vi "LabJSONExample.vi"(8 "Error In":errorcluster, 9 "Settings":T1, 10 "JSON Input":string="{\n  \"Cluster\":{\n    \"Numeric\":1,\n    \"String\":\"One\",\n    \"Checkbox\":false\n  },\n  \"Array - String\":[[]],\n  \"Numeric\":0,\n  \"File Path Control\":\"\",\n  \"Checkbox\":false\n}", 11 "VI Path":path=path "Sample/SampleVI.vi") -> (0 "Error Out":errorcluster, 3 "JSON Output":string)   [LabVIEW 2019, in "LabJSON.lvlib"]
doc: "Take JSON as input, run the VI, and return the output as JSON"
uses:
  LabJSON.lvlib
  Typedefs/Settings.ctl
  <vilib>/SLL Toolkit/SLL File IO/SLL File IO.lvlib
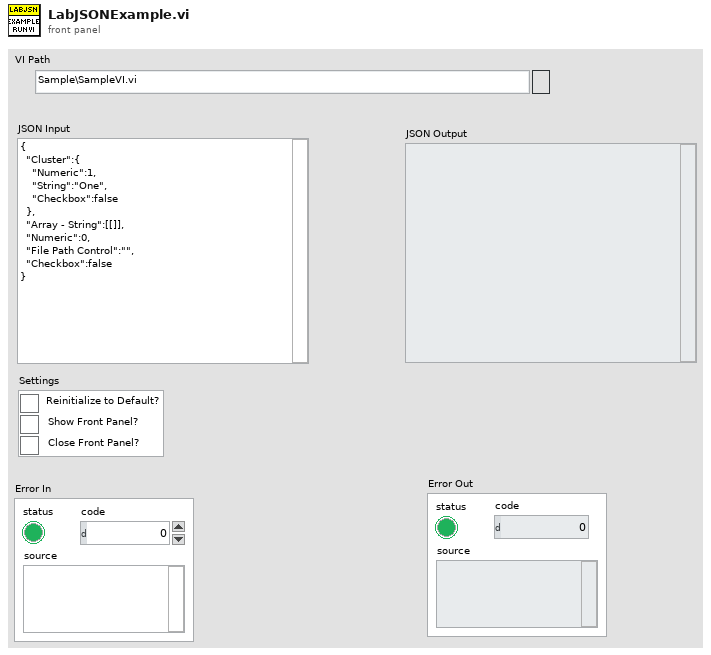
[diagram p1: front panel]
types:
  T1 = typedef "LabJSON.lvlib/Settings.ctl" = cluster{"Reinitialize to Default?":bool, "Show Front Panel?":bool, "Close Front Panel?":bool}
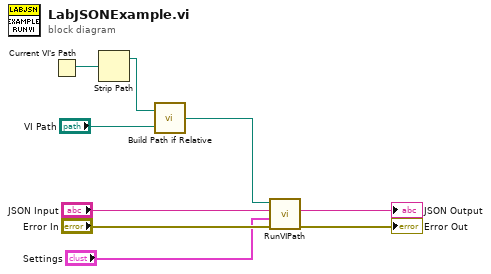
[diagram p0: block diagram]
diagram:
  n1 = Current VI's Path() -> (path=w8:path)
  n2 = Strip Path(path=w8) -> (stripped path=w7:path)  [unwired: 1 out]
  n3 = call <vilib>:"Build Path if Relative.vi"("Relative or Absolute Path"="VI Path", "Base Path"=w7) -> ("Path Out"=w6:path)
  n4 = call "RunVIPath.vi"("Error In"="Error In", "Settings"="Settings", "JSON Input"="JSON Input", "VI Path"=w6) -> ("Error Out"=→"Error Out":errorcluster, "JSON Output"=→"JSON Output":string)  [unwired: 6 in]
